vi "FieldPost.vi"(7 "CC Cycles":i32=10, 8 "error in (no error)":errorcluster, 11 "comms cluster in":T1={600, 49682, "Modbus master out"=refnum}) -> (0 "error out":errorcluster={"status"=FALSE, "code"=0, "source"="Post passed -- System successfully initialised"}, 3 "comms cluster out":T1={600, 49682, "Modbus master out"=refnum})   [LabVIEW 2025]
uses:
  <vilib>/Modbus/master/Modbus Master.lvclass
  <vilib>/Modbus/subvis/Transmission Data Unit (ADU)/IP Data Unit/IP Data Unit.lvclass
  <vilib>/Modbus/subvis/Protocol/TCP/TCP Master/TCP Master.lvclass
panel:
  in  "Required Pass (%)":i32=80
  # "Post Panel I/O\n\nPerforms pre-cycle testing of physical\nI/O connection from server. LabVIEW\nnatively handles errors as a result of \nserver communication loss, however, \ncommunication between server and\nfield I/O can fail. Server keeps watch-\ndog for each field I/O. This subVI \nchecks watchdog for \"CC cycles\" \nnumber of communication cycles \nif there is \"Required Pass (%)\" %\nsuccess rate of frame transfers \ncycle will begin, else, subVI\nwill return failure and program will \nhalt\n\nINPUTS:\n  1. comms cluster input of:\n      a) station reg start address\n      b)16-bit modulo of local user IP\n      c) MB comms line \n  2. error line in.\n  3. CC Cycles - number of pre-check \n      cycles to determine pass\nOUTPUTS:\n  1. comms cluster out of:\n      a) station reg start address\n      b)16-bit modulo of local user IP\n      c) MB comms line \n   2. error line out"
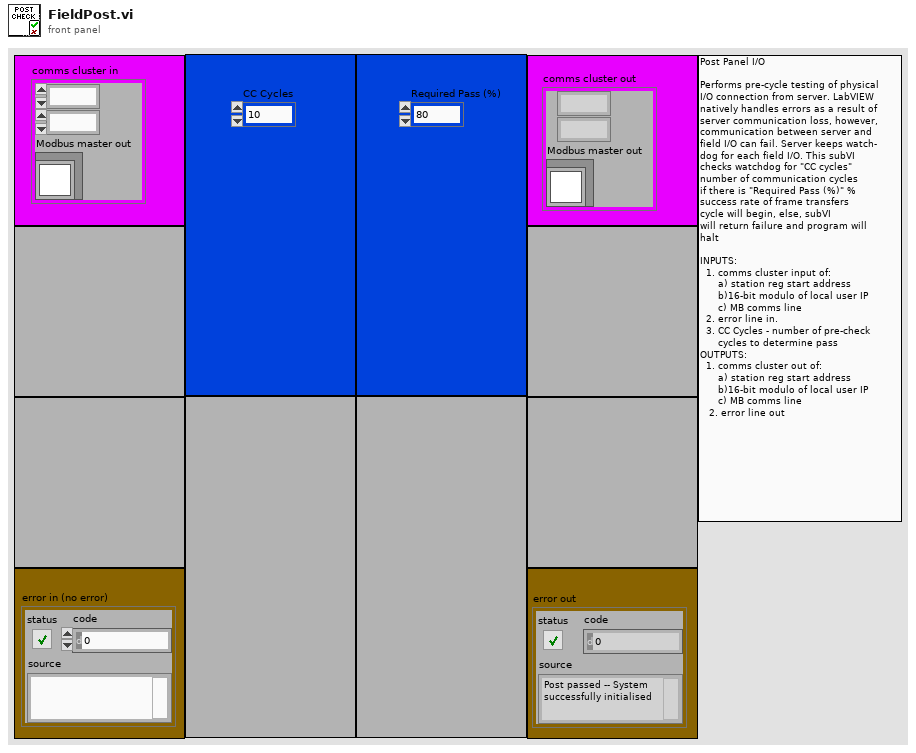
[diagram p1: front panel]
types:
  T1 = cluster{u16, u32, "Modbus master out":refnum<class "Modbus Master.lvclass">}
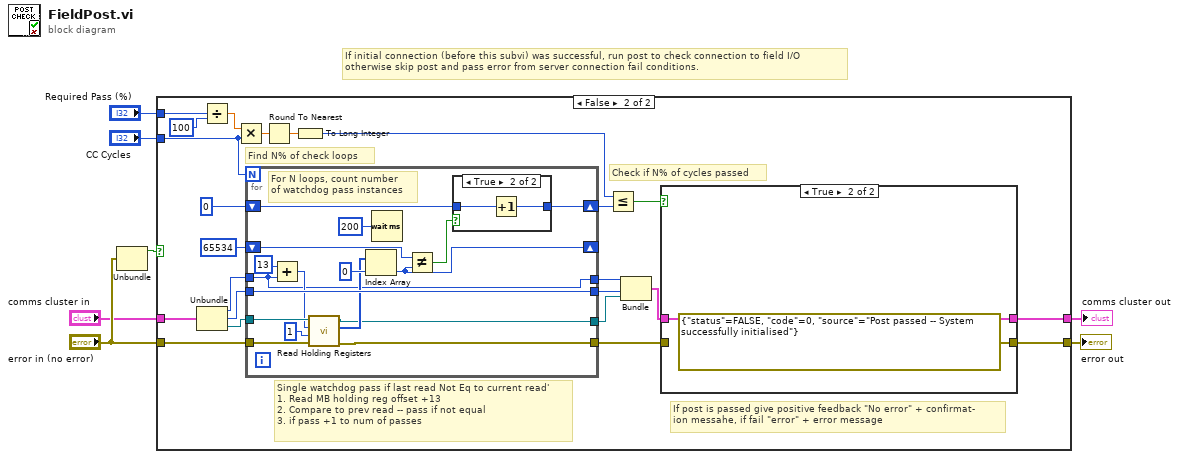
[diagram p0: block diagram]
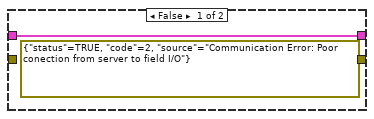
[diagram p3: hidden frame]
diagram:
  # "If initial connection (before this subvi) was successful, run post to check connection to field I/O\notherwise skip post and pass error from server connection fail conditions."
  n1 = Unbundle("error in (no error)") -> ("status"=w6:bool)  [unwired: 2 out]
  n2 = case shown="False" w6 {
    tunnel: "error in (no error)" -> [w8 w32]
    tunnel: "comms cluster in" -> [w9 w31]
    tunnel: [w9 w24] -> w3
    tunnel: "CC Cycles" -> [_ w14]
    tunnel: [w8 w17] -> w7
    tunnel: "Required Pass (%)" -> [_ w12]
    frame True {
    }
    frame False {
      # "If post is passed give positive feedback \"No error\" + confirmat-\nion messahe, if fail \"error\" + error message"
      # "Check if N% of cycles passed"
      # "Single watchdog pass if last read Not Eq to current read'\n1. Read MB holding reg offset +13\n2. Compare to prev read -- pass if not equal\n3. if pass +1 to num of passes"
      # "Find N% of check loops"
      n3 = Unbundle(w31) -> (w30:u16, w29:u32, "Modbus master out"=w28:refnum<class "Modbus Master.lvclass">)
      n4 = Divide(x=w12, y=100) -> (x/y=w10:dbl)
      n5 = Multiply(x=w10, y=w14) -> (x*y=w16:dbl)
      n6 = for {
        N: w14 -> [_]
        tunnel: w32 -> [w52]
        tunnel: w30 -> [w38]
        tunnel: w29 -> [w51]
        tunnel: w28 -> [w53]
        shift-right: [w43] -> _
        shift-left: u16 65534 -> [w45]
        tunnel: [w51] -> w19
        shift-right: [w41] -> w23
        shift-left: u16 0 -> [w42]
        tunnel: [w40] -> w20
        tunnel: [w39] -> w25
        tunnel: [w38] -> w21
        # "For N loops, count number\nof watchdog pass instances"
        n7 = Add(x=u16 13, y=w38) -> (x+y=w49:u16)
        n8 = call-dynamic "Read Holding Registers.vi"("error in (no error)"=w52, "number of holding registers"=u16 1, "starting address"=w49, "Modbus master in"=w53) -> ("error out"=w39:errorcluster, "register values"=w46:u16[], "Modbus master out"=w40:refnum<class "Modbus Master.lvclass">)  [unwired: 5 in]
        n9 = Index Array(array=w46, index=0) -> (element=w43:u16)
        n10 = Wait (ms)(milliseconds to wait=u32 200) -> ()  [unwired: 1 out]
        n11 = Not Equal?(x=w45, y=w43) -> (x != y?=w44:bool)
        n12 = case shown="True" w44 {
          tunnel: w42 -> [w54 w56]
          tunnel: [w54 w55] -> w41
          frame False {
          }
          frame True {
            n13 = Increment(x=w56) -> (x+1=w55:u16)
          }
        }
      }
      n14 = Round To Nearest(number=w16) -> (nearest integer value=w15:dbl)
      n15 = To Long Integer(number=w15) -> (32bit integer=w13:i32)
      n16 = Less Or Equal?(x=w13, y=w23) -> (x <= y?=w22:bool)
      n17 = Bundle(w21, w19, "Modbus master out"=w20) -> (w18:T1)  [unwired: 1 in]
      n18 = case shown="True" w22 {
        tunnel: w25 -> [_ _]
        tunnel: [w34 w36] -> w24
        tunnel: w18 -> [w34 w36]
        tunnel: [errorcluster {"status"=TRUE, "code"=2, "source"="Communication Error: Poor conection from server to field I/O"} ("error out") errorcluster {"status"=FALSE, "code"=0, "source"="Post passed -- System successfully initialised"} ("error out")] -> w17
        frame False {
        }
        frame True {
        }
      }
    }
  }
  "error out" <- w7
  "comms cluster out" <- w3
